vi "lv_server.vi"() -> ()   [LabVIEW 2018]
doc: "This WebSockets API example VI acts as a server for an incoming websockets connection. Receives/sends string data to the connected client.\nWebSockets 2.0.0.38\nSam Sharp - MediaMongrels Ltd\nCopyright (c) 2019, MediaMongrels Ltd"
uses:
  <vilib>/MediaMongrels Ltd/WebSockets/Sockets/VISA TCP Listener/VISA TCP Listener.lvclass
  <vilib>/MediaMongrels Ltd/WebSockets/WebSockets/WebSocket Server/WebSocket Server.lvclass
  <vilib>/wsapi/NI_WebServices.lvlib
  <vilib>/Analysis/NI_AALBase.lvlib
panel:
  in  "Send img":bool
  in  "Stop":bool
  out "Received Data":string
  in  "Send":bool
  in  "Data":string
  # "WebSockets Server Example"
  # "This VI is a simple example of sending/receiving data using WebSockets.\nIt waits for a single incoming WebSockets connection on Port 6123 and\nthen displays incoming string data. Strings can also be sent back to the client.\n\nInstructions for use:\n1) Run this VI\n2) Open the index.html file located in the examples folder or the 'Client Single Connection' example or deploy the 'Test Client' web service and visiting the web service URL\n3) The index.html will display the status of the connection and once established, data can be sent/received from either this VI or the index.html file.\n\nNote: For Microsoft Edge, you may need to access the index.html file by first deploying the 'Test Client' Web Service, executing \"CheckNetIsolation LoopbackExempt -a -n=Microsoft.MicrosoftEdge_8wekyb3d8bbwe\" to enable WebSockets on a loopback and then visiting http://localhost:<web service port>/index.html"
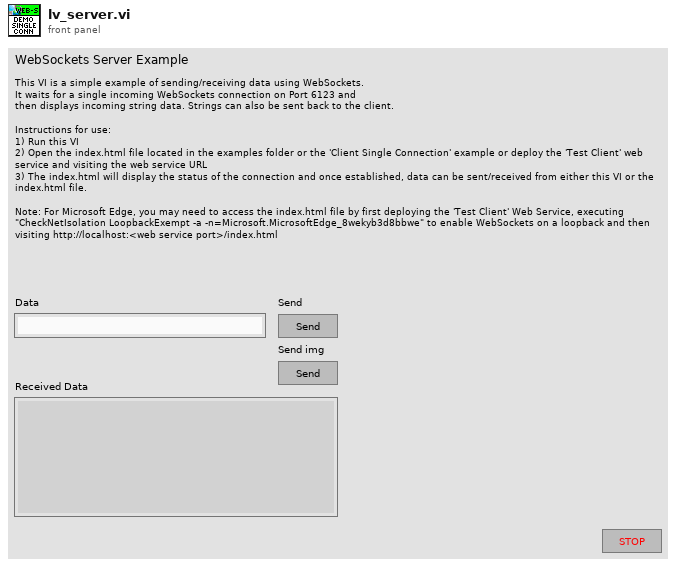
[diagram p1: front panel]
types:
  T1 = typedef "imagedata.ctl" = cluster{"image type":i32, "image depth":i32, "image":u8[], "mask":u8[], "colors":u32[], "Rectangle":cluster{"left":i16, "top":i16, "right":i16, "bottom":i16}}
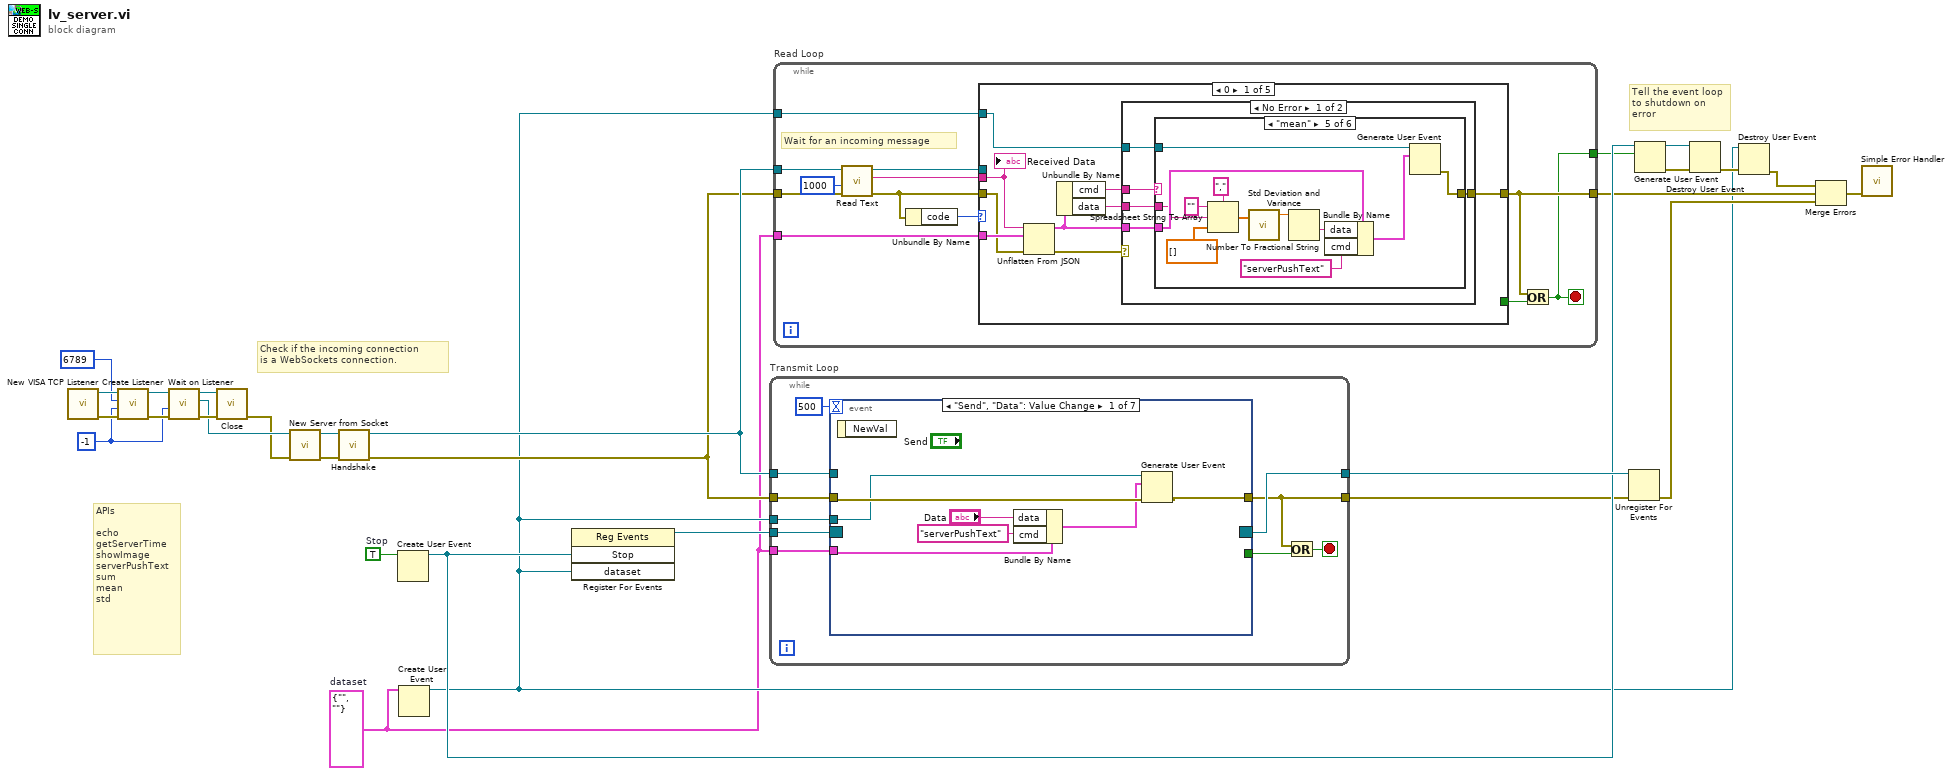
[diagram p0: block diagram]
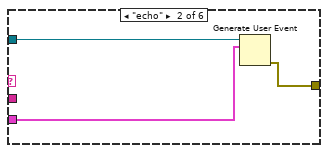
[diagram p3: hidden frame]
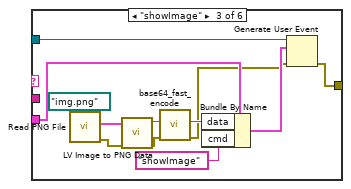
[diagram p4: hidden frame]
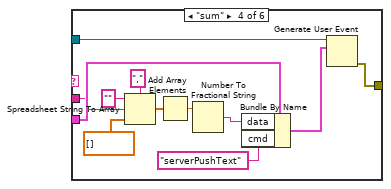
[diagram p5: hidden frame]
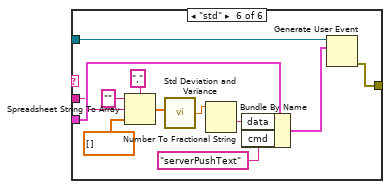
[diagram p6: hidden frame]
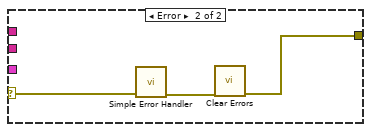
[diagram p7: hidden frame]
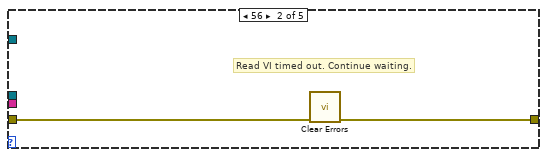
[diagram p8: hidden frame]
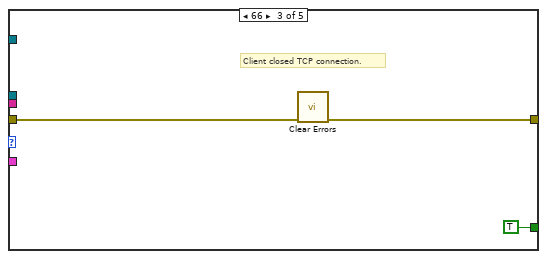
[diagram p9: hidden frame]
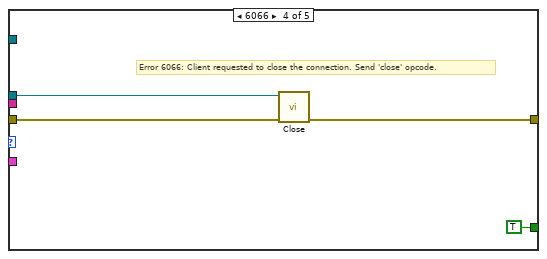
[diagram p10: hidden frame]
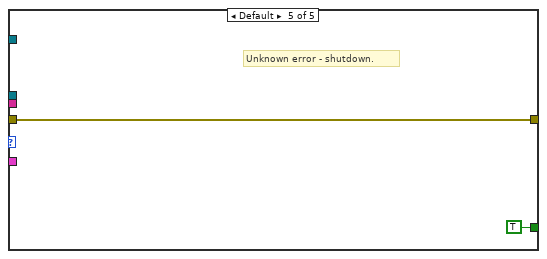
[diagram p11: hidden frame]
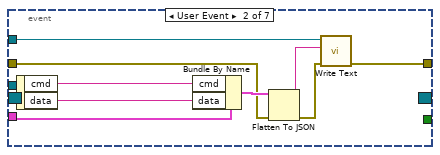
[diagram p12: hidden frame]
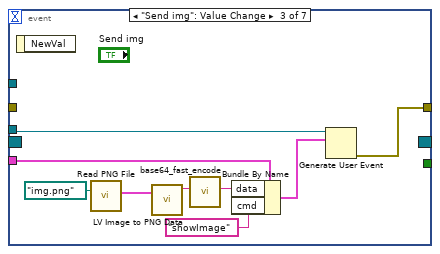
[diagram p13: hidden frame]
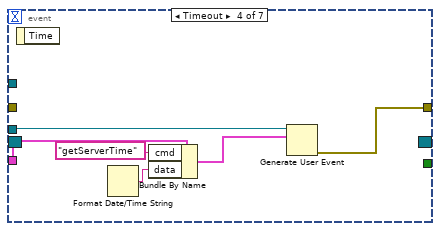
[diagram p14: hidden frame]
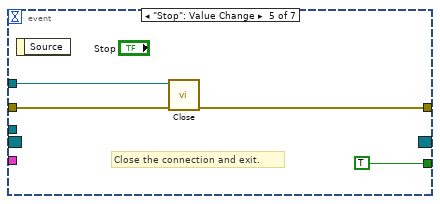
[diagram p15: hidden frame]
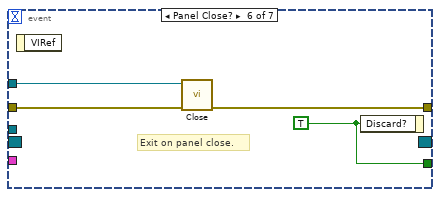
[diagram p16: hidden frame]
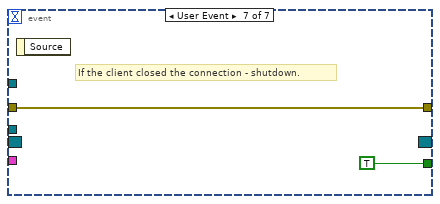
[diagram p17: hidden frame]
diagram:
  w1 = cluster{"cmd":string, "data":string} {"cmd"="", "data"=""}  # dataset
  w28 = TRUE  # Stop
  w9 = -1 ("timeout ms (25000)")
  # "APIs\n\necho\ngetServerTime\nshowImage\nserverPushText\nsum\nmean\nstd"
  # "Tell the event loop to shutdown on error"
  # "Check if the incoming connection\nis a WebSockets connection."
  n1 = call <vilib>:"New VISA TCP Listener.vi"() -> ("error out"=w15:errorcluster, "VISA TCP Listener out"=w16:refnum<class "VISA TCP Listener.lvclass">)  [unwired: 10 in]
  n2 = call-dynamic "Create Listener.vi"("error in (no error)"=w15, "timeout ms (5000)"=w9, "Port"=u16 6789 ("port"), "VISA TCP Listener in"=w16) -> ("error out"=w13:errorcluster, "VISA TCP Listener out"=w11:refnum<class "VISA TCP Listener.lvclass">)  [unwired: 6 in]
  n3 = call-dynamic "Wait on Listener.vi"("error in (no error)"=w13, "timeout ms (5000)"=w9, "VISA TCP Listener in"=w11) -> ("error out"=w14:errorcluster, "Socket out"=w8:refnum<class "Socket.lvclass">, "VISA TCP Listener out"=w12:refnum<class "VISA TCP Listener.lvclass">)  [unwired: 6 in]
  n4 = call-dynamic "Close.vi"("error in (no error)"=w14, "VISA TCP Listener in"=w12) -> ("error out"=w7:errorcluster)  [unwired: 9 in]
  n5 = call <vilib>:"New Server from Socket.vi"("error in (no error)"=w7, "Socket"=w8) -> ("error out"=w17:errorcluster, "WebSocket Server out"=w18:refnum<class "WebSocket Server.lvclass">)  [unwired: 8 in]
  n6 = call-dynamic "Handshake.vi"("error in (no error)"=w17, "WebSocket Connection in"=w18) -> ("error out"=w3:errorcluster, "WebSocket Connection out"=w4:refnum<class "WebSocket Server.lvclass">)  [unwired: 8 in]
  n7 = Create User Event(user event datatype=w28) -> (user event=w26:refnum<user-event>)  [unwired: 1 in, 1 out]
  n8 = Create User Event(user event datatype=w1) -> (user event=w2:refnum<user-event>)  [unwired: 1 in, 1 out]
  n9 = register-events(w26, w2) -> (reference out=w29:refnum<event-registration>)  [unwired: 2 in, 1 out]
  n10 = while "Transmit Loop" {
    tunnel: w4 -> [w39]
    tunnel: w29 -> [w38]
    tunnel: [w37] -> w27
    tunnel: [w33] -> w21
    tunnel: w3 -> [w36]
    tunnel: w1 -> [w32]
    tunnel: w2 -> [w30]
    stop <- w34 stop-if-true
    n11 = event shown="[0] \"Send\", \"Data\": Value Change" {
      selector: w38 -> [_ _ _ _ _ _ _]
      dyn-events: [_ _ _ _ _ _ _] -> w37
      timeout: 500 -> [_ _ _ _ _ _ _]
      tunnel: w39 -> [_ w55 _ _ w73 w78 _]
      tunnel: [_ _ _ _ TRUE w77 TRUE] -> w35
      tunnel: [w43 w54 w56 w65 w72 w76 w79] -> w33
      tunnel: w36 -> [w42 w48 _ _ w71 w75 w79]
      tunnel: w32 -> [w44 w52 w61 w69 _ _ _]
      tunnel: w30 -> [w41 _ w58 w70 _ _ _]
      event "Send", "Data": Value Change {
        n12 = event-data() -> ()  [unwired: 1 in, 1 out]
        n13 = Bundle By Name(cluster=w44, "data"="Data", "cmd"="serverPushText" ("state")) -> (w40:cluster{"cmd":string, "data":string})
        n14 = Generate User Event(user event=w41, event data cluster=w40, error in=w42) -> (error out=w43:errorcluster)  [unwired: 1 in, 1 out]
      }
      event User Event {
        n15 = event-data() -> ("cmd"=w50:string, "data"=w49:string)  [unwired: 1 in]
        n16 = Bundle By Name(cluster=w52, "cmd"=w50, "data"=w49) -> (w53:cluster{"cmd":string, "data":string})
        n17 = Flatten To JSON(anything=w53, error in (no error)=w48) -> (JSON string=w51:string, 11:w47:errorcluster)  [unwired: 1 in]
        n18 = call-dynamic "Write Text.vi"("error in (no error)"=w47, "String Data"=w51, "WebSocket in"=w55) -> ("error out"=w54:errorcluster)  [unwired: 7 in, 1 out]
      }
      event "Send img": Value Change {
        n19 = event-data() -> ()  [unwired: 1 in, 1 out]
        n20 = call <vilib>:"Read PNG File.vi"("path to PNG file"=path "img.png") -> ("image data"=w64:T1)  [unwired: 8 in, 2 out]
        n21 = call <vilib>:"LV Image to PNG Data.vi"("image data"=w64) -> ("png data"=w63:string)  [unwired: 9 in, 1 out]
        n22 = call "base64_fast_encode.vi"("string in (not encoded)"=w63) -> ("string out (base64-encoded)"=w60:string)  [unwired: 9 in, 1 out]
        n23 = Bundle By Name(cluster=w61, "data"=w60, "cmd"="showImage" ("state")) -> (w57:cluster{"cmd":string, "data":string})
        n24 = Generate User Event(user event=w58, event data cluster=w57) -> (error out=w56:errorcluster)  [unwired: 2 in, 1 out]
      }
      event Timeout {
        n25 = event-data() -> ()  [unwired: 1 in, 1 out]
        n26 = Format Date/Time String() -> (date/time string=w66:string)  [unwired: 3 in]
        n27 = Bundle By Name(cluster=w69, "cmd"="getServerTime", "data"=w66) -> (w68:cluster{"cmd":string, "data":string})
        n28 = Generate User Event(user event=w70, event data cluster=w68) -> (error out=w65:errorcluster)  [unwired: 2 in, 1 out]
      }
      event "Stop": Value Change {
        # "Close the connection and exit."
        n29 = event-data() -> ()  [unwired: 1 in, 1 out]
        n30 = call-dynamic "Close.vi"("error in (no error)"=w71, "WebSocket in"=w73) -> ("error out"=w72:errorcluster)  [unwired: 9 in]
      }
      event Panel Close? {
        w77 = TRUE ("Discard?")
        # "Exit on panel close."
        n31 = event-data() -> ()  [unwired: 1 in, 1 out]
        n32 = call-dynamic "Close.vi"("error in (no error)"=w75, "WebSocket in"=w78) -> ("error out"=w76:errorcluster)  [unwired: 9 in]
        n33 = event-data("Discard?"=w77) -> ()  [unwired: 1 in, 1 out]
      }
      event User Event {
        # "If the client closed the connection - shutdown."
        n34 = event-data() -> ()  [unwired: 1 in, 1 out]
      }
    }
    n35 = Or(x=w33, y=w35) -> (x .or. y?=w34:bool)
  }
  n36 = while "Read Loop" {
    tunnel: w4 -> [w92]
    tunnel: [w83] -> w25
    tunnel: [w85] -> w20
    tunnel: w3 -> [w86]
    tunnel: w2 -> [w82]
    tunnel: w1 -> [w81]
    stop <- w83 stop-if-true
    # "Wait for an incoming message"
    n37 = call-dynamic "Read Text.vi"("error in (no error)"=w86, "timeout ms (5000)"=1000 ("timeout ms (25000)"), "WebSocket in"=w92) -> ("error out"=w87:errorcluster, "Data"=w89:string, "WebSocket out"=w88:refnum<class "WebSocket Server.lvclass">)  [unwired: 6 in]
    n38 = Unbundle By Name(w87) -> ("code"=w90:i32)
    n39 = case shown="0" w90 {
      tunnel: w89 -> [w101 _ _ _ _]
      tunnel: [_ _ TRUE TRUE TRUE] -> w84
      tunnel: w88 -> [_ _ _ w169 _]
      tunnel: w87 -> [w99 w162 w164 w167 w170]
      tunnel: [w97 w161 w163 w166 w170] -> w85
      tunnel: w82 -> [w94 _ _ _ _]
      tunnel: w81 -> [w100 _ _ _ _]
      frame 0 {
        n40 = Unflatten From JSON(JSON string=w101, type and defaults=w100, error in (no error)=w99) -> (value=w93:cluster{"cmd":string, "data":string}, error out=w98:errorcluster)  [unwired: 4 in]
        n41 = Unbundle By Name(w93) -> ("cmd"=w96:string, "data"=w95:string)
        n42 = case shown="No Error" w98 {
          selector: w98 -> [_ w159]
          tunnel: [w102 w160] -> w97
          tunnel: w96 -> [w106 _]
          tunnel: w95 -> [w105 _]
          tunnel: w94 -> [w104 _]
          tunnel: w93 -> [w103 _]
          frame No Error {
            n43 = case shown="\"mean\"" w106 {
              tunnel: w105 -> [_ _ _ w127 w139 w151]
              tunnel: w104 -> [_ w109 w116 w132 w144 w156]
              tunnel: w103 -> [_ w108 w113 w129 w141 w153]
              tunnel: [_ w107 w115 w131 w143 w155] -> w102
              frame "False", Default {
              }
              frame "echo" {
                n44 = Generate User Event(user event=w109, event data cluster=w108) -> (error out=w107:errorcluster)  [unwired: 2 in, 1 out]
              }
              frame "showImage" {
                n45 = call <vilib>:"Read PNG File.vi"("path to PNG file"=path "img.png") -> ("error out"=w112:errorcluster, "image data"=w121:T1)  [unwired: 8 in, 1 out]
                n46 = call <vilib>:"LV Image to PNG Data.vi"("error in (no error)"=w112, "image data"=w121) -> ("error out"=w111:errorcluster, "png data"=w120:string)  [unwired: 8 in]
                n47 = call "base64_fast_encode.vi"("error in (no error)"=w111, "string in (not encoded)"=w120) -> ("error out"=w110:errorcluster, "string out (base64-encoded)"=w118:string)  [unwired: 8 in]
                n48 = Bundle By Name(cluster=w113, "data"=w118, "cmd"="showImage" ("state")) -> (w114:cluster{"cmd":string, "data":string})
                n49 = Generate User Event(user event=w116, event data cluster=w114, error in=w110) -> (error out=w115:errorcluster)  [unwired: 1 in, 1 out]
              }
              frame "sum" {
                n50 = Spreadsheet String To Array(delimiter (Tab)=",", format string="", spreadsheet string=w127, array type (2D Dbl)=dbl[] []) -> (array=w125:dbl[])
                n51 = Add Array Elements(numeric array=w125) -> (sum=w124:dbl)
                n52 = Number To Fractional String(number=w124) -> (F-format string=w123:string)  [unwired: 3 in]
                n53 = Bundle By Name(cluster=w129, "data"=w123, "cmd"="serverPushText" ("state")) -> (w130:cluster{"cmd":string, "data":string})
                n54 = Generate User Event(user event=w132, event data cluster=w130) -> (error out=w131:errorcluster)  [unwired: 2 in, 1 out]
              }
              frame "mean" {
                n55 = Spreadsheet String To Array(delimiter (Tab)=",", format string="", spreadsheet string=w139, array type (2D Dbl)=dbl[] []) -> (array=w135:dbl[])
                n56 = call <vilib>:"Std Deviation and Variance.vi"("X"=w135) -> ("mean"=w134:dbl)  [unwired: 1 in, 2 out]
                n57 = Number To Fractional String(number=w134) -> (F-format string=w137:string)  [unwired: 3 in]
                n58 = Bundle By Name(cluster=w141, "data"=w137, "cmd"="serverPushText" ("state")) -> (w142:cluster{"cmd":string, "data":string})
                n59 = Generate User Event(user event=w144, event data cluster=w142) -> (error out=w143:errorcluster)  [unwired: 2 in, 1 out]
              }
              frame "std" {
                n60 = Spreadsheet String To Array(delimiter (Tab)=",", format string="", spreadsheet string=w151, array type (2D Dbl)=dbl[] []) -> (array=w147:dbl[])
                n61 = call <vilib>:"Std Deviation and Variance.vi"("X"=w147) -> ("standard deviation"=w146:dbl)  [unwired: 1 in, 2 out]
                n62 = Number To Fractional String(number=w146) -> (F-format string=w149:string)  [unwired: 3 in]
                n63 = Bundle By Name(cluster=w153, "data"=w149, "cmd"="serverPushText" ("state")) -> (w154:cluster{"cmd":string, "data":string})
                n64 = Generate User Event(user event=w156, event data cluster=w154) -> (error out=w155:errorcluster)  [unwired: 2 in, 1 out]
              }
            }
          }
          frame Error {
            n65 = call <vilib>:"Simple Error Handler.vi"("error in (no error)"=w159) -> ("error out"=w158:errorcluster)  [unwired: 4 in, 4 out]
            n66 = call <vilib>:"Clear Errors.vi"("error in (no error)"=w158) -> ("error out"=w160:errorcluster)  [unwired: 5 in, 1 out]
          }
        }
        "Received Data" <- w101
      }
      frame 56 {
        # "Read VI timed out. Continue waiting."
        n67 = call <vilib>:"Clear Errors.vi"("error in (no error)"=w162) -> ("error out"=w161:errorcluster)  [unwired: 5 in, 1 out]
      }
      frame 66 {
        # "Client closed TCP connection."
        n68 = call <vilib>:"Clear Errors.vi"("error in (no error)"=w164) -> ("error out"=w163:errorcluster)  [unwired: 5 in, 1 out]
      }
      frame 6066 {
        # "Error 6066: Client requested to close the connection. Send 'close' opcode."
        n69 = call-dynamic "Close.vi"("error in (no error)"=w167, "WebSocket in"=w169) -> ("error out"=w166:errorcluster)  [unwired: 9 in]
      }
      frame Default {
        # "Unknown error - shutdown."
      }
    }
    n70 = Or(x=w85, y=w84) -> (x .or. y?=w83:bool)
  }
  n71 = Unregister For Events(event registration refnum=w27, error in=w21) -> (error out=w19:errorcluster)
  n72 = Generate User Event(user event=w26, event data cluster=w25) -> (user event out=w24:refnum<user-event>, error out=w23:errorcluster)  [unwired: 2 in]
  n73 = Destroy User Event(user event=w24, error in=w23) -> (error out=w6:errorcluster)
  n74 = Destroy User Event(user event=w2, error in=w6) -> (error out=w5:errorcluster)
  n75 = Merge Errors(w5, w20, w19) -> (w22:errorcluster)
  n76 = call <vilib>:"Simple Error Handler.vi"("error in (no error)"=w22) -> ()  [unwired: 4 in, 5 out]
